vi "Or77200_SetActPos.vi"(8 "ErrorIn(No Error)":errorcluster caption="entrée d'erreur (pas d'erreur)", 11 "Port":refnum<visa-resource-name>) -> (0 "sortie d'erreur":errorcluster, 3 "Port Out":refnum<visa-resource-name>)   [LabVIEW 2010]
uses:
  <vilib>/Utility/config.llb/Write Key (Double).vi
  <vilib>/Utility/config.llb/NI_LVConfig.lvlib
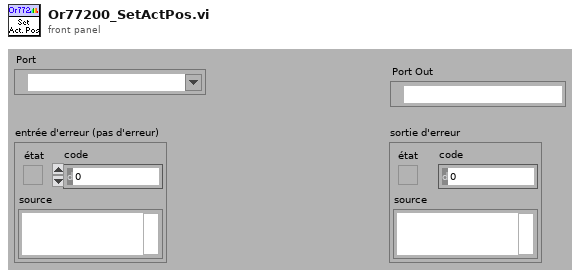
[diagram p1: front panel]
types:
  T1 = typedef "NI_LVConfig.lvlib/Config Data RefNum.ctl" = refnum<k1>
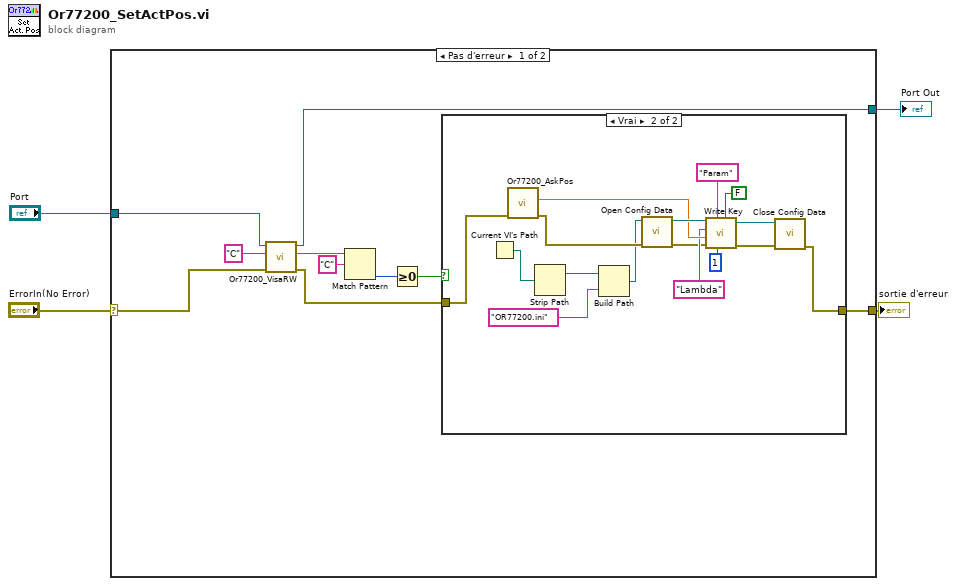
[diagram p0: block diagram]
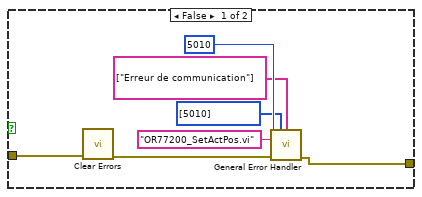
[diagram p2: hidden frame]
diagram:
  n1 = case shown="Pas d'erreur" "ErrorIn(No Error)" {
    selector: "ErrorIn(No Error)" -> [w8 w39]
    tunnel: [w14 w39] -> w3
    tunnel: "Port" -> [w7 w38]
    tunnel: [w5 w38] -> w1
    frame No Error {
      n2 = call <userlib>:"Or77200_VisaRW.vi"("error in"=w8, "Commande"="C", "Port"=w7) -> ("error out"=w6:errorcluster, "Response"=w12:string, "Port Out"=w5:refnum<visa-resource-name>)  [unwired: 5 in, 1 out]
      n3 = Match Pattern(string=w12, regular expression="C" ("x")) -> (offset past match=w11:i32)  [unwired: 1 in, 3 out]
      n4 = Greater Or Equal To 0?(x=w11) -> (x >= 0?=w9:bool)
      n5 = case shown="Vrai" w9 {
        tunnel: [w15 w23] -> w14
        tunnel: w6 -> [w16 w22]
        frame False {
          n6 = call <vilib>:"Clear Errors.vi"("error in (no error)"=w16) -> ("error out"=w21:errorcluster)  [unwired: 6 in]
          n7 = call <vilib>:"General Error Handler.vi"("[error code] (0)"=5010, "[user-defined codes]"=i32[] [5010], "[user-defined descriptions]"=string[] ["Erreur de communication"], "[error source] (\" \")"="OR77200_SetActPos.vi" ("[error source] (\" \")"), "error in (no error)"=w21) -> ("error out"=w15:errorcluster)  [unwired: 6 in, 4 out]
        }
        frame True {
          n8 = Current VI's Path() -> (path=w31:path)
          n9 = call <userlib>:"Or77200_AskPos.vi"("error In"=w22) -> ("sortie d'erreur"=w32:errorcluster, "Lambda Out"=w36:dbl)  [unwired: 9 in]
          n10 = Strip Path(path=w31) -> (stripped path=w30:path)  [unwired: 1 out]
          n11 = Build Path(base path=w30, name or relative path="OR77200.ini" ("nom ou chemin relatif")) -> (appended path=w28:path)
          n12 = call <vilib>:"Open Config Data.vi"("error in (no error)"=w32, "configuration file path"=w28) -> ("error out"=w33:errorcluster, "refnum"=w37:T1)  [unwired: 7 in, 1 out]
          n13 = call-poly <vilib>:"Write Key.vi"("use system decimal point (T)"=FALSE, "precision (6)"=i16 1, "section"="Param", "error in (no error)"=w33, "value"=w36, "key"="Lambda", "refnum"=w37) -> ("error out"=w25:errorcluster, "refnum out"=w24:T1)  [unwired: 2 in, 1 out]
          n14 = call <vilib>:"Close Config Data.vi"("error in (no error)"=w25, "refnum"=w24) -> ("error out"=w23:errorcluster)  [unwired: 8 in, 1 out]
        }
      }
    }
    frame Error {
    }
  }
  "sortie d'erreur" <- w3
  "Port Out" <- w1
